vi "Kontroll Interferent changed.vi"(10 "Kontroll-Interferent:":u16, 11 "Kontroll-Interferent: alt":u16) -> (3 "geändert":bool)   [LabVIEW 2020, in "EPA 1065.lvlib" / "HovaCAL Interference verificaton.lvlib"]
uses:
  HovaCAL Interference verificaton.lvlib
  Aktion Index uebersetzten.ctl
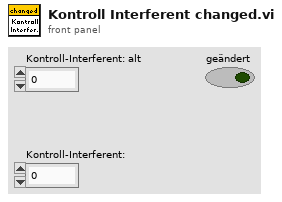
[diagram p1: front panel]
types:
  T1 = typedef "EPA 1065.lvlib/HovaCAL Interference verificaton.lvlib/Aktion Index uebersetzten.ctl" = enum16{"lesen", "schreiben", "auswerten", "Referenzwert", "KompIndex", "RefInterferIndex", "KontrInterfIndex"}
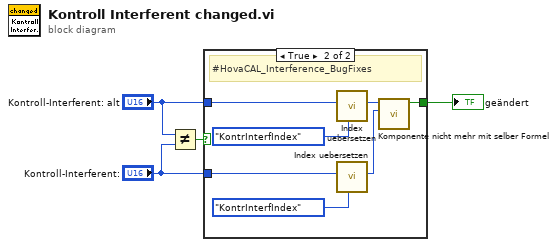
[diagram p0: block diagram]
diagram:
  n1 = Not Equal?(x="Kontroll-Interferent: alt", y="Kontroll-Interferent:") -> (x != y?=w1:bool)
  n2 = case shown="True" w1 {
    tunnel: [_ w7] -> w4
    tunnel: "Kontroll-Interferent: alt" -> [_ w6]
    tunnel: "Kontroll-Interferent:" -> [_ w5]
    frame False {
    }
    frame True {
      # "#HovaCAL_Interference_BugFixes"
      n3 = call "Index uebersetzen.vi"("Aktion"=Aktion_Index_uebersetzten."KontrInterfIndex", "Index relativ:"=w6) -> ("Index absolut"=w11:i32)  [unwired: 4 in, 5 out]
      n4 = call "Index uebersetzen.vi"("Aktion"=Aktion_Index_uebersetzten."KontrInterfIndex", "Index relativ:"=w5) -> ("Index absolut"=w9:i32)  [unwired: 4 in, 5 out]
      n5 = call "Komponente nicht mehr mit selber Formel.vi"("neue Komponente"=w9, "alte Kompomente"=w11) -> ("geändert"=w7:bool)  [unwired: 9 in]
    }
  }
  "geändert" <- w4
